vi "RVC Drive to Point Maneuver.vi"() -> ()   [LabVIEW 2014]
uses:
  <vilib>/Simulation/Scripting/Companion Diagram/SimConfigNode/SimParams.ctl
  <vilib>/Simulation/Scripting/Companion Diagram/SimConfigNode/_simSolvers.ctl
  <vilib>/Simulation/Implementation/Shared/SIMSCR Execution Mode.ctl
  <vilib>/Platform/TimedLoop/XDataNode/timing_clust.ctl
  <vilib>/Platform/TimedLoop/XDataNode/nitl_modes.ctl
  <vilib>/Platform/TimedLoop/XDataNode/wakeup.ctl
  <vilib>/Simulation/Param Hierarchy/Typedefs/SIMPH Param Control Actions.ctl
  <vilib>/Simulation/Scripting/Editor Utilities/SIM subVI tag data.ctl
  <vilib>/Simulation/Scripting/Editor Utilities/SIM subVI execution type.ctl
  <vilib>/Simulation/Implementation/Shared/NILVSim_ParamChanged.vi
  <vilib>/Simulation/Implementation/Shared/NILVSim_FinishedLate.vi
  <vilib>/Simulation/Implementation/Shared/NILVSIM_BeginStep.vi
  <vilib>/Simulation/Utility/Implementation/SIM Time.vi
  <vilib>/Simulation/Utility/Implementation/NILVSim Collector.llb/SIM Collector (vector).vi
  <vilib>/Simulation/Utility/Implementation/SIM Halt.vi
  <vilib>/Simulation/SignalArithmetic/Implementation/NILVSim Gain.llb/SIM Gain (scalar).vi
  <vilib>/Analysis/coordinate.llb/Wrap Angle.vi
  <vilib>/Analysis/coordinate.llb/Wrap Angle (scalar).vi
  <vilib>/Simulation/Implementation/Shared/SIM Fire Discrete SubVI.vi
  <vilib>/Simulation/Implementation/Shared/NILVSim_Manager.vi
  <vilib>/Utility/error.llb/Clear Errors.vi
  <vilib>/Simulation/Implementation/Shared/NILVSim_FinalizeModel.vi
  <vilib>/Simulation/Utility/Implementation/NILVSim Collector.llb/NILVSim Collector core (vector).vi
  <vilib>/Simulation/Implementation/Shared/SIM Fire Discrete SubVI (Core).vi
  <vilib>/Simulation/Implementation/Shared/SIM Unbundle Sim Info.vi
  <vilib>/Simulation/Implementation/Shared/SIMSH Read Queue.vi
  <vilib>/Simulation/Implementation/Shared/NILVSim_Initialize.vi
  <vilib>/Simulation/Utility/Implementation/NILVSim Get Time and IsAcceptedStep.vi
  subVIs/2D Animate Rotating Wheel.vi
  subVIs/2D Animation Plot.vi
  <vilib>/Simulation/Implementation/Shared/NILVSim_GetModelError.vi
  <vilib>/Simulation/Implementation/Shared/SIM Bundle Sim Info.vi
  <vilib>/Simulation/Scripting/Companion Diagram/SimConfigNode/SimDog.xnode
  SIM Bicycle.vi
  <vilib>/Platform/TimedLoop/XDataNode/XDataNode.xnode
  <vilib>/Simulation/Implementation/XNodeFramework/SimXNode/SimX.xnode
  <vilib>/Analysis/NI_AAL_Angle.lvlib
  <vilib>/Platform/TimedLoop/XDataNode/XDNodeRunTimeDep.lvlib
  <vilib>/Simulation/Implementation/Shared/NI_SIM_Implementation.lvlib
panel:
  out "Coordinate Frame":cluster{dbl[], dbl[]}[](graph)
  out "velocity":dbl(knob)=1.0 scale=0.0..2.0
  out "XY Graph - Drive to Point":cluster{"Time":dbl[], "Signal":dbl[]}[](graph)
  out "Position":cluster{"x":dbl, "y":dbl, "theta":dbl}
  out "Steering Angle":dbl format="%.2f"
  out "Steering Angle":picture
  in  "Goal":dbl[](array[numeric])=[5.0, 5.0]
  # "Velocity"
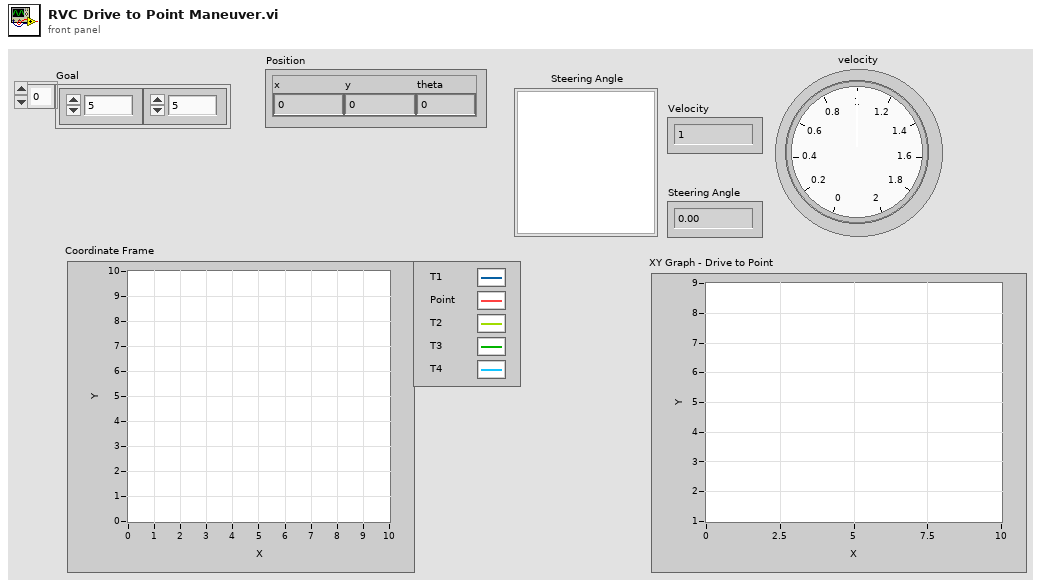
[diagram p1: front panel]
types:
  T1 = typedef "SIMSCR Execution Mode.ctl" = enum16{"Simulate to Completion", "Single Time-Step Simulation (Fixed Step Only)"}
  T2 = typedef "XDNodeRunTimeDep.lvlib/timing_clust.ctl" = cluster{"Expected End [f-1]":u64, "Actual End [f-1]":u64, "Finished Late? [f-1]":bool, "Expected End [i-1]":u64, "Actual End [i-1]":u64, "Finished Late? [i-1]":bool, "Expected Start [i]":u64, "Actual Start [i]":u64, "Expected Start [f]":u64, "Actual Start [f]":u64, "Source Name":string, "Structure Name":string, "Period":i64, "Deadline":i64, "Offset":i64, "Start":i64, "Priority":i32, "Timeout":i32, "Mode":T3, "Wakeup Reason":T4, "Error":errorcluster, "Source Type":string, "Secondary Source Type":string, "Global End Time":u64, "Global Start Time":u64, "Frame Duration":u64, "Iteration Duration":u64, "Assigned CPU":i32, "I/O Scan Engine Mode":u32}
  T3 = typedef "XDNodeRunTimeDep.lvlib/nitl_modes.ctl" = enum32{"No Change", "Process missed periods, maintain original phase", "Discard missed periods, maintain original phase", "Process missed periods, ignore original phase", "Discard missed periods, ignore original phase"}
  T4 = typedef "XDNodeRunTimeDep.lvlib/wakeup.ctl" = enum32{"Normal", "Aborted", "Asynchronous wakeup", "Timing source error", "Timed loop error", "Timeout"}
  T5 = typedef "SIMPH Param Control Actions.ctl" = enum16{"get params", "set params"}
  T6 = typedef "SIM subVI tag data.ctl" = cluster{"period":dbl, "skew":dbl, "Simulation execution type":T7}
  T7 = typedef "SIM subVI execution type.ctl" = enum16{"Function call", "Discrete", "Continuous", "Initialization only", "Final step only"}
  T8 = cluster{"SIMSH Sim Time":dbl, "Build Array 2":cluster{"appended array":dbl[]}, "Divide 2":cluster{"x/y":dbl}, "Sine & Cosine":cluster{"sin(x)":dbl, "cos(x)":dbl}, "initial condition":dbl[], "Index Array 4":cluster{"element":dbl}, "vel limit":cluster{"output":dbl}, "steering angle limit":cluster{"output":dbl}, "acceleration limit":cluster{"output":dbl}, "Product":cluster{"Result":dbl[]}, "Build Array":cluster{"appended array":dbl[]}, "Integrator":cluster{"output":dbl[]}}
  T9 = typedef "SimParams.ctl" = cluster{"Initial Time (s)":dbl, "Final Time (s)":dbl, "Step Size (s)":dbl, "ODE Solver":T10, "Minimum Step Size (s)":dbl, "Maximum Step Size (s)":dbl, "Relative Tolerance":dbl, "Absolute Tolerance":dbl, "Software Timing":bool, "Initial Step Size (s)":dbl, "Automatic Fixed Step Size?":bool, "Automatic Discrete Step Size?":bool, "Discrete Step Size (s)":dbl, "Calculate using Time Step":bool, "Solver Wired?":bool, "Prev.Frm.Expected End":u64, "Prev.Frm.Actual End":u64, "Prev.Frm.Finished Late?":bool, "Prev.Iter.Expected End":u64, "Prev.Iter.Actual End":u64, "Prev.Iter.Finished Late?":bool, "Expected Iteration Start":u64, "Actual Iteration Start":u64, "Expected Frame Start":u64, "Actual Frame Start":u64, "Source Name":string, "Name":string, "Period":i64, "Deadline":i64, "Offset":i64, "Start":i64, "Priority":i32, "Timeout":i32, "Processor":i32, "Mode":enum32{"No Change", "Process missed periods, maintain original phase", "Discard missed periods, maintain original phase", "Process missed periods, ignore original phase", "Discard missed periods, ignore original phase"}, "Wakeup reason":enum32{"Normal", "Aborted", "Asynchronous wakeup", "Timing source error", "Timed loop error", "Timeout"}, "Error":errorcluster, "Source Type":string, "Secondary Source Type":string, "Global End Time":u64, "Global Start Time":u64, "Full Solver Reset":bool, "Execution Mode":T1, "Nan/Inf Check":bool, "Custom Solver Library":string, "Solver Is Variable":bool, "custom solver name":string, "Signal Collection Decimation":u32}
  T10 = typedef "_simSolvers.ctl" = enum16{"Runge-Kutta 1 (Euler)", "Runge-Kutta 2", "Runge-Kutta 3", "Runge-Kutta 4", "Runge-Kutta 23 (variable)", "Runge-Kutta 45 (variable)", "BDF (variable)", "Adams-Moulton (variable)", "Rosenbrock (variable)", "Discrete States Only", "SDIRK 4 (variable)", "Radau 5 (variable)", "Radau 9 (variable)", "Radau 13 (variable)", "Radau [Variable Order] (variable)", "Gear's Method (variable)", "Linearizer", "State Query", "Trim Eval", "Custom Solver"}
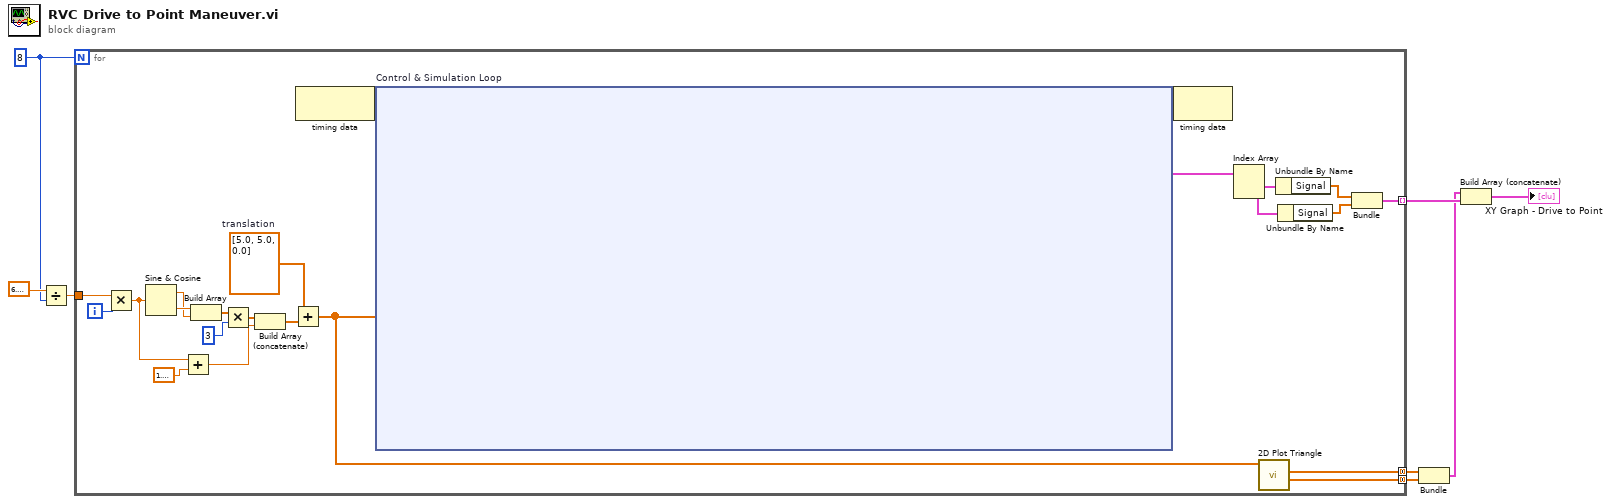
[diagram p0: block diagram]
diagram:
  w6 = 8
  n1 = Divide(x=6.283185307179586, y=w6) -> (x/y=w5:dbl)
  n2 = for {
    N: w6 -> [_]
    tunnel: [w22] -> w8 mode=indexing
    tunnel: w5 -> [w18]
    tunnel: [w13] -> w3 mode=concatenating
    tunnel: [w12] -> w2 mode=concatenating
    i -> [w19]
    w9 = dbl[] [5.0, 5.0, 0.0]  # translation
    n3 = Multiply(x=w18, y=w19) -> (x*y=w14:dbl)
    n4 = Sine & Cosine(0:w14) -> (1:w20:dbl, 2:w21:dbl)
    n5 = Add(x=w14, y=1.5707963267948966) -> (x+y=w11:dbl)
    n6 = Build Array(w21, w20) -> (w29:dbl[])
    n7 = Multiply(x=w29, y=3) -> (x*y=w28:dbl[])
    n8 = Build Array (concatenate)(w28, w11) -> (w15:dbl[])
    n9 = Add(x=w9, y=w15) -> (x+y=w10:dbl[])
    n10 = node-c288() -> (w31:variant)  [unwired: 1 in]
    n11 = node-c254 "Control & Simulation Loop"(w31, w10) -> (w30:variant, w27:cluster{"Time":dbl[], "Signal":dbl[]}[])
    n12 = node-c288(w30) -> ()  [unwired: 1 out]
    n13 = Index Array(array=w27) -> (element #1=w26:cluster{"Time":dbl[], "Signal":dbl[]}, element #2=w25:cluster{"Time":dbl[], "Signal":dbl[]})  [unwired: 2 in]
    n14 = call "2D Plot Triangle.vi"("appended array"=w10) -> ("Y"=w12:dbl[], "X"=w13:dbl[])  [unwired: 8 in, 1 out]
    n15 = Unbundle By Name(w26) -> ("Signal"=w24:dbl[])
    n16 = Unbundle By Name(w25) -> ("Signal"=w23:dbl[])
    n17 = Bundle("Signal"=w24, "Signal"=w23) -> (w22:cluster{"Signal":dbl[], "Signal":dbl[]})  [unwired: 1 in]
  }
  n18 = Bundle("X"=w3, "Y"=w2) -> (w1:cluster{"X":dbl[], "Y":dbl[]})  [unwired: 1 in]
  n19 = Build Array (concatenate)(w1, w8) -> (→"XY Graph - Drive to Point":cluster{"Signal":dbl[], "Signal":dbl[]}[])
